vi "Write Data To Instrument.vi"(8 "error in (no error)":errorcluster, 9 "File (\"INT:\\UserData.txt\")":string="INT:\\UserData.txt", 10 "Data (\"hello\")":string="hello", 11 "VISA resource name":refnum<visa-resource-name>) -> (0 "error out":errorcluster, 3 "VISA resource name out":refnum<visa-resource-name>)   [LabVIEW 2017, in "Agilent 3352X Series.lvlib"]
doc: "Writes specific data to a local file in file system stored in non-volatile memory ( the instrument memory or an external USB memory)"
uses:
  Doppia_Freq_Circuito/Agilent 3352X Series/Agilent 3352X Series.lvlib
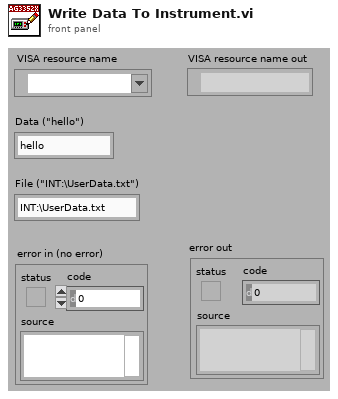
[diagram p1: front panel]
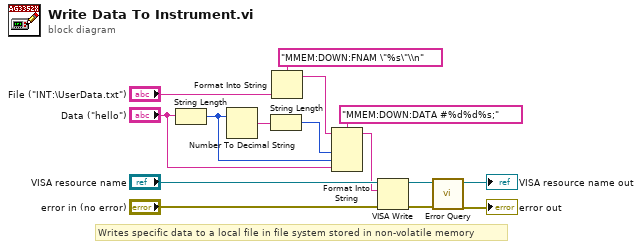
[diagram p0: block diagram]
diagram:
  # "Writes specific data to a local file in file system stored in non-volatile memory"
  n1 = String Length(string="Data (\"hello\")") -> (length=w5:i32)
  n2 = Number To Decimal String(number=w5) -> (decimal integer string=w4:string)  [unwired: 1 out]
  n3 = String Length(string=w4) -> (length=w3:i32)
  n4 = Format Into String(format string="MMEM:DOWN:FNAM \"%s\"\\n", "File (\"INT:\\UserData.txt\")") -> (resulting string=w1:string)  [unwired: 2 in, 1 out]
  n5 = Format Into String(format string="MMEM:DOWN:DATA #%d%d%s;", initial string=w1, w3, w5, "Data (\"hello\")") -> (resulting string=w2:string)  [unwired: 1 in, 1 out]
  n6 = VISA Write(VISA resource name="VISA resource name", write buffer=w2, error in (no error)="error in (no error)") -> (VISA resource name out=w10:refnum<visa-resource-name>, error out=w9:errorcluster)  [unwired: 1 out]
  n7 = call "Error Query.vi"("error in (no error)"=w9, "VISA resource name"=w10) -> ("error out"=→"error out":errorcluster, "VISA resource name out"=→"VISA resource name out":refnum<visa-resource-name>)  [unwired: 8 out]
